vi "test2.vi"() -> ()   [LabVIEW 2013]
uses:
  LightField Automation.lvclass
panel:
  in  "On Chip Accumulations 2":i32
  out "On Chip Accumulations":i32
  in  "Intensifier Gain":i32=1
  in  "ExperimentName":string="Experiment2"
  in  "?":bool
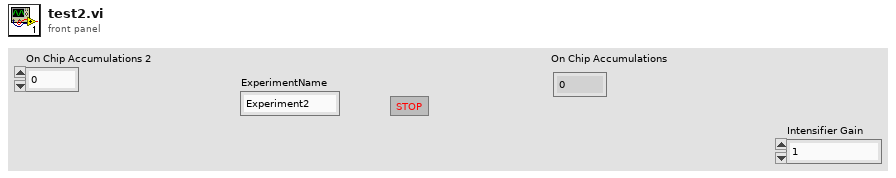
[diagram p1: front panel]
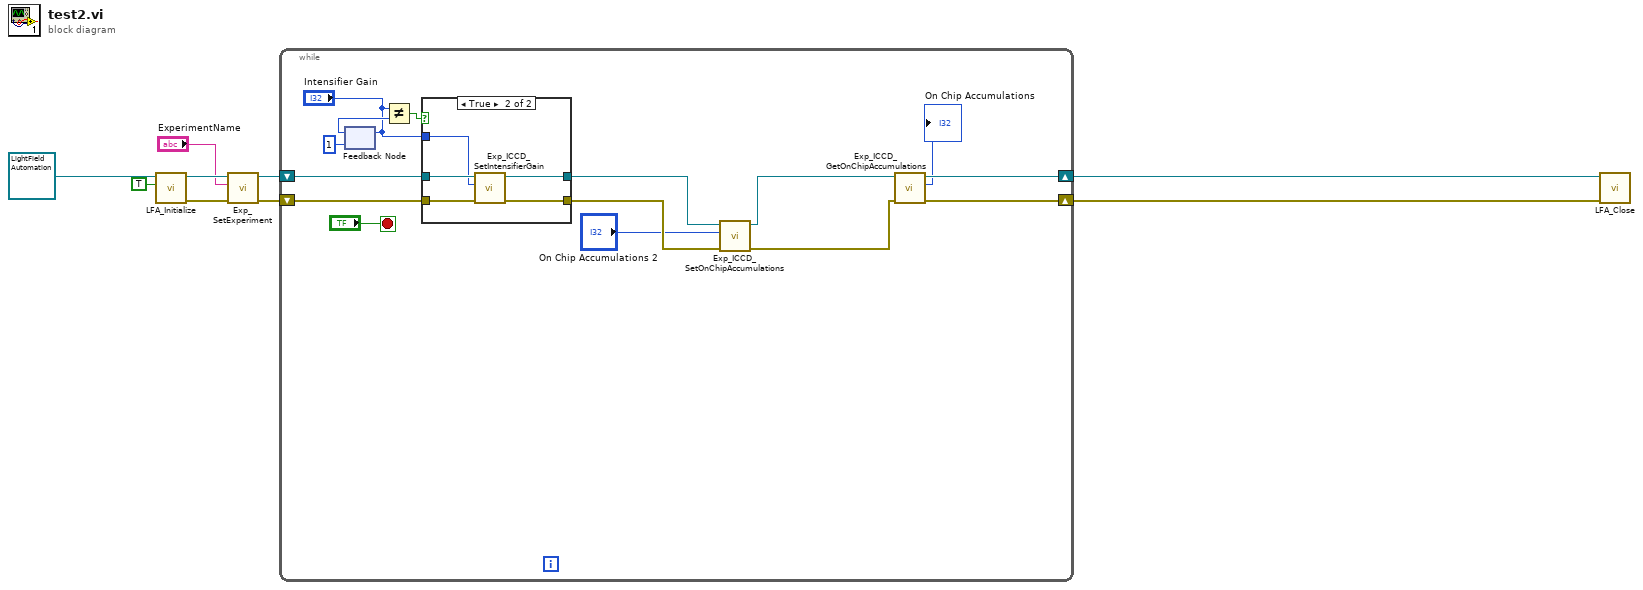
[diagram p0: block diagram]
diagram:
  n1 = call "LFA_Initialize.vi"("Is Visible?"=TRUE, "LightField Automation in"=refnum<class "LightField Automation.lvclass"> refnum ("LightField Automation.lvclass")) -> ("error out"=w6:errorcluster, "LightField Automation out"=w7:refnum<class "LightField Automation.lvclass">)  [unwired: 8 in]
  n2 = call "Exp_SetExperiment.vi"("error in (no error)"=w6, "ExperimentName"="ExperimentName", "LightField Automation in"=w7) -> ("error out"=w5:errorcluster, "LightField Automation out"=w4:refnum<class "LightField Automation.lvclass">)  [unwired: 7 in]
  n3 = while {
    shift-right: [w16] -> w2
    shift-left: w4 -> [w21]
    shift-right: [w17] -> w1
    shift-left: w5 -> [w20]
    stop <- "?" stop-if-true
    n4 = feedback #1(1 ("Intensifier Gain")) -> (w23:i32)
    n5 = feedback-in #1("Intensifier Gain") -> ()
    n6 = Not Equal?(x="Intensifier Gain", y=w23) -> (x != y?=w22:bool)
    n7 = case shown="True" w22 {
      tunnel: "Intensifier Gain" -> [_ w27]
      tunnel: w21 -> [w25 w31]
      tunnel: w20 -> [w26 w30]
      tunnel: [w25 w28] -> w14
      tunnel: [w26 w29] -> w13
      frame False {
      }
      frame True {
        n8 = call "Exp_ICCD_SetIntensifierGain.vi"("error in (no error)"=w30, "Intensifier Gain"=w27, "LightField Automation in"=w31) -> ("error out"=w29:errorcluster, "LightField Automation out"=w28:refnum<class "LightField Automation.lvclass">)  [unwired: 7 in]
      }
    }
    n9 = call "Exp_ICCD_SetOnChipAccumulations.vi"("error in (no error)"=w13, "On Chip Accumulations"="On Chip Accumulations 2", "LightField Automation in"=w14) -> ("error out"=w11:errorcluster, "LightField Automation out"=w12:refnum<class "LightField Automation.lvclass">)  [unwired: 7 in]
    n10 = call "Exp_ICCD_GetOnChipAccumulations.vi"("error in (no error)"=w11, "LightField Automation in"=w12) -> ("error out"=w17:errorcluster, "On Chip Accumulations"=→"On Chip Accumulations":i32, "LightField Automation out"=w16:refnum<class "LightField Automation.lvclass">)  [unwired: 7 in]
  }
  n11 = call "LFA_Close.vi"("error in (no error)"=w1, "LightField Automation in"=w2) -> ()  [unwired: 8 in, 2 out]
